vi "GEOM_SortDetectors.vi"(10 "Detectors":T1 {"ReadModes"."amplifiers"."fliped" items=["none", "horizontal", "vertical"]; "ReadModes"."amplifiers"."type" items=["LL", "LR", "UL", "UR"]}) -> (2 "Sorted Detectors":T1 {"ReadModes"."amplifiers"."fliped" items=["none", "horizontal", "vertical"]; "ReadModes"."amplifiers"."type" items=["LL", "LR", "UL", "UR"]})   [LabVIEW 2016]
uses:
  GEOM_FPADetectors.ctl
  GEOM_DetStruct.ctl
  GEOM_ReadMode.ctl
  GEOM_Amplifier.ctl
  GEOM_AmpType.ctl
  GEOM_ROI.ctl
  GEOM_Coords.ctl
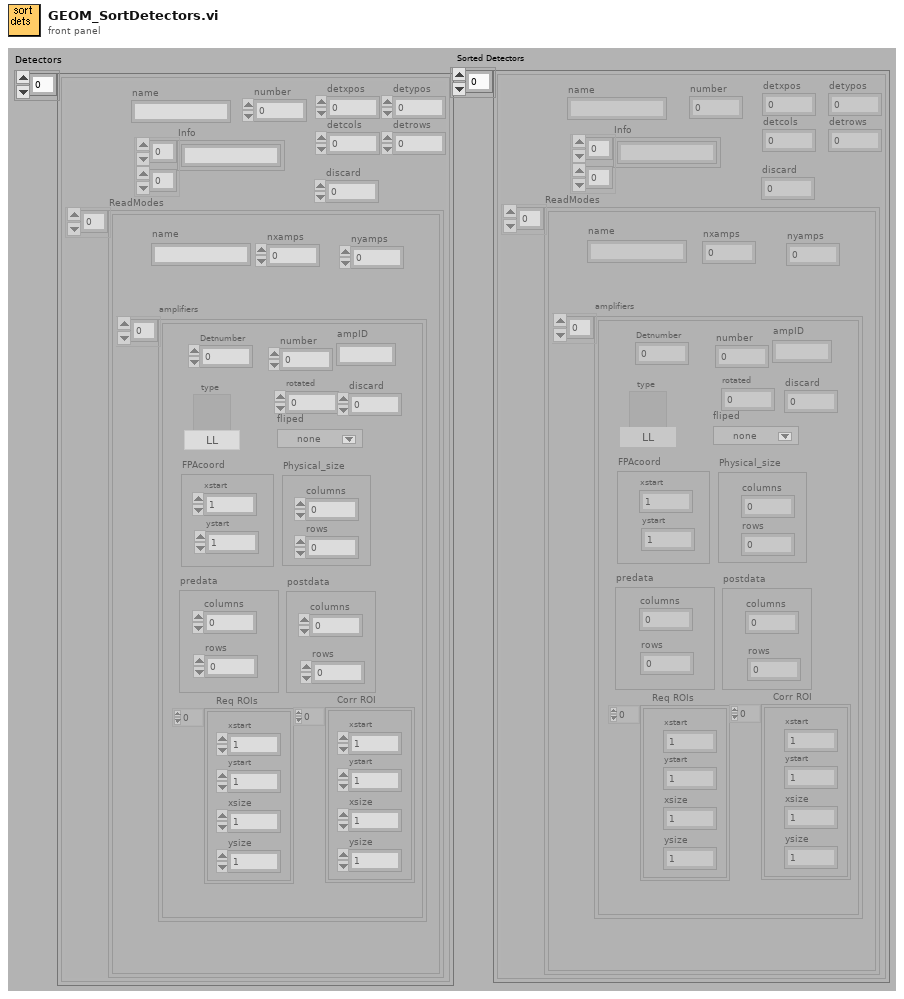
[diagram p1: front panel]
types:
  T1 = typedef "GEOM_FPADetectors.ctl" = T2[]
  T2 = typedef "GEOM_DetStruct.ctl" = cluster{"name":string, "number":i32, "Info":string[][], "ReadModes":T3[], "detxpos":i32, "detypos":i32, "detcols":i32, "detrows":i32, "discard":i32}
  T3 = typedef "GEOM_ReadMode.ctl" = cluster{"name":string, "amplifiers":T4[], "nxamps":i32, "nyamps":i32}
  T4 = typedef "GEOM_Amplifier.ctl" = cluster{"number":i32, "type":T5, "rotated":i16, "fliped":u16, "FPAcoord":cluster{"xstart":i32, "ystart":i32}, "Physical_size":cluster{"columns":i32, "rows":i32}, "predata":cluster{"columns":i32, "rows":i32}, "postdata":cluster{"columns":i32, "rows":i32}, "Req ROIs":T6, "Corr ROI":T6, "Detnumber":i32, "ampID":string, "discard":i32}
  T5 = typedef "GEOM_AmpType.ctl" = u16
  T6 = typedef "GEOM_ROI.ctl" = T7[]
  T7 = typedef "GEOM_Coords.ctl" = cluster{"xstart":u32, "ystart":u32, "xsize":u32, "ysize":u32}
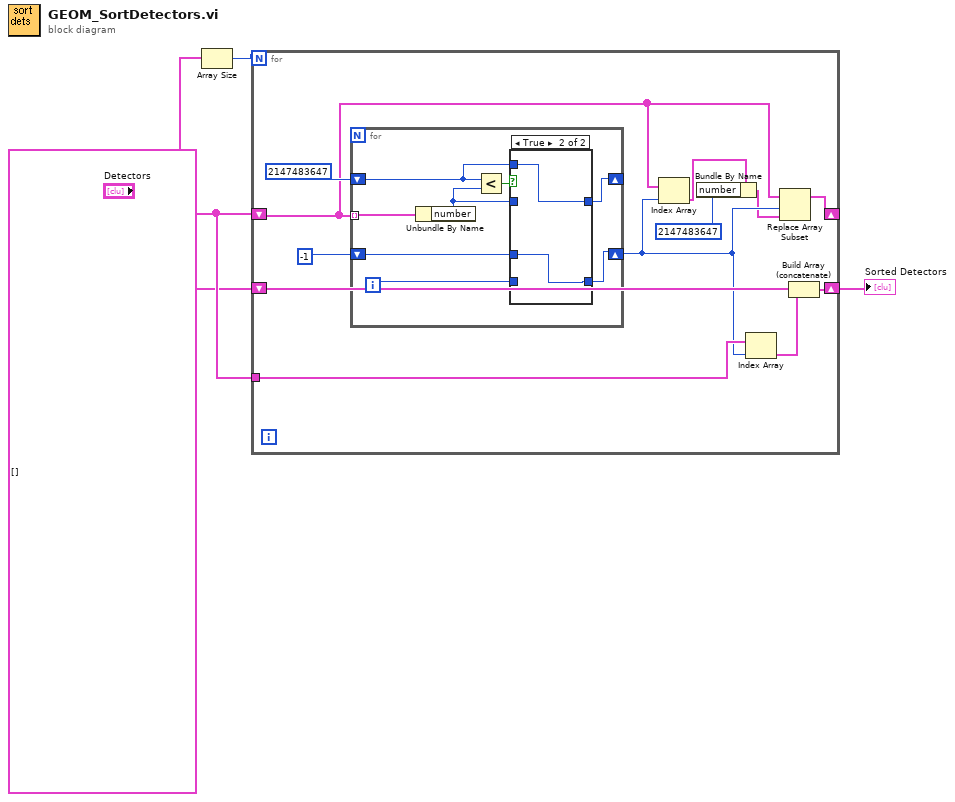
[diagram p0: block diagram]
diagram:
  n1 = Array Size(array="Detectors") -> (size(s)=w4:i32)
  n2 = for {
    N: w4 -> [_]
    shift-right: [w10] -> _
    shift-left: "Detectors" -> [w8]
    shift-right: [w12] -> w2
    shift-left: T2[] [] -> [w11]
    tunnel: "Detectors" -> [w14]
    n3 = for {
      shift-right: [w20] -> _
      shift-left: 2147483647 -> [w19]
      tunnel: w8 -> [w24] mode=indexing
      shift-right: [w18] -> w9
      shift-left: -1 -> [w17]
      i -> [w22]
      n4 = Unbundle By Name(w24) -> ("number"=w21:i32)
      n5 = Less?(x=w19, y=w21) -> (x < y?=w23:bool)
      n6 = case shown="True" w23 {
        tunnel: w22 -> [w25 _]
        tunnel: w21 -> [w26 _]
        tunnel: [w26 w28] -> w20
        tunnel: w19 -> [_ w28]
        tunnel: [w25 w27] -> w18
        tunnel: w17 -> [_ w27]
        frame False {
        }
        frame True {
        }
      }
    }
    n7 = Index Array(array=w8, index=w9) -> (element=w7:T2)
    n8 = Bundle By Name(cluster=w7, "number"=2147483647) -> (w6:T2)
    n9 = Index Array(array=w14, index=w9) -> (element=w13:T2)
    n10 = Replace Array Subset(array=w8, new element=w6, index=w9) -> (w10:T1)
    n11 = Build Array (concatenate)(w11, w13) -> (w12:T2[])
  }
  "Sorted Detectors" <- w2
